vi "lxw version id.vi"(8 "error in (no error)":errorcluster) -> (0 "error out":errorcluster, 3 "function return":u16)   [LabVIEW 8.6]
doc: "uint16_t lxw_version_id(void);"
uses:
  pending_lvxlsxwriter/xlsxwriter.dll
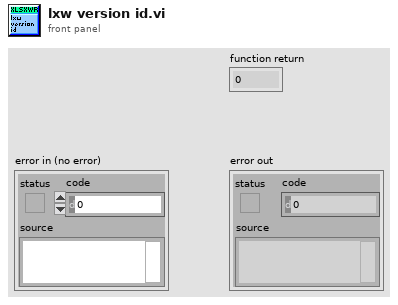
[diagram p1: front panel]
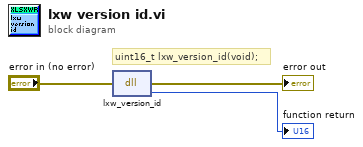
[diagram p0: block diagram]
diagram:
  # "uint16_t lxw_version_id(void);"
  n1 = dll-call lib="C:/Users/WDAGUtilityAccount/Desktop/pending_lvxlsxwriter/xlsxwriter.*" fn="lxw_version_id"(error in="error in (no error)") -> (error out=→"error out":errorcluster, →"function return":u16)  [unwired: 2 in, 1 out]
